vi "TCP client test.vi"() -> ()   [LabVIEW 2014]
panel:
  out "x-y":u32
  out "毫秒计时值":u32
  out "长度":i32
  out "服务器消息":string
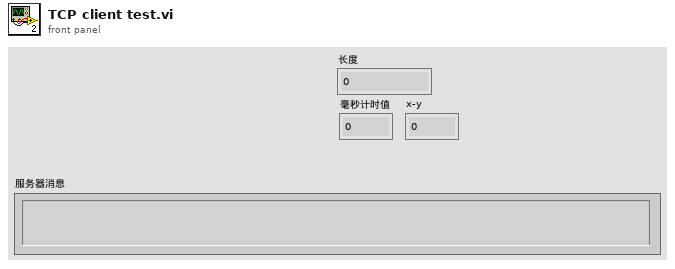
[diagram p1: front panel]
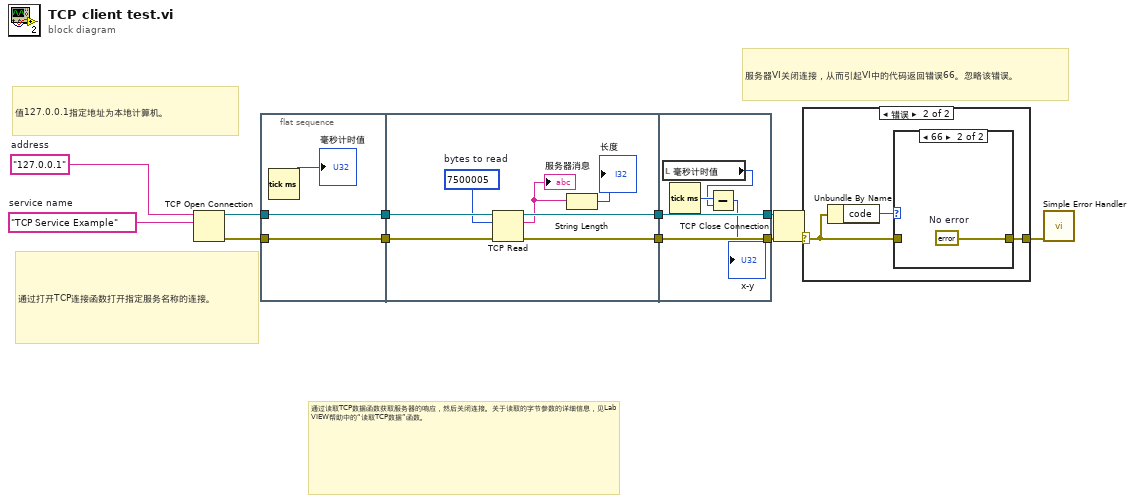
[diagram p0: block diagram]
diagram:
  w7 = "TCP Service Example"  # service name
  w8 = "127.0.0.1"  # address
  # "服务器VI关闭连接，从而引起VI中的代码返回错误66。忽略该错误。"
  # "值127.0.0.1指定地址为本地计算机。"
  # "通过打开TCP连接函数打开指定服务名称的连接。"
  # "通过读取TCP数据函数获取服务器的响应，然后关闭连接。关于读取的字节参数的详细信息，见LabVIEW帮助中的“读取TCP数据”函数。"
  n1 = TCP Open Connection(address=w8, remote port or service name=w7) -> (connection ID=w11:refnum<k5>, error out=w12:errorcluster)  [unwired: 3 in]
  n2 = flat-sequence {
    tunnel: w11 -> [w14]
    tunnel: w12 -> [w15]
    tunnel: [w15] -> w4
    tunnel: [w14] -> w3
    tunnel: w4 -> [w22]
    tunnel: w3 -> [w21]
    tunnel: [w20] -> w2
    tunnel: [w19] -> w1
    tunnel: [w26] -> w9
    tunnel: [w27] -> w10
    tunnel: w2 -> [w27]
    tunnel: w1 -> [w26]
    frame #0 {
      n3 = Tick Count (ms)() -> (millisecond timer value=→"毫秒计时值":u32)
    }
    frame #1 {
      w18 = 7500005  # bytes to read
      n4 = TCP Read(connection ID=w21, bytes to read=w18, error in (no error)=w22) -> (connection ID out=w20:refnum<k5>, data out=w17:string, error out=w19:errorcluster)  [unwired: 2 in]
      "服务器消息" <- w17
      n5 = String Length(string=w17) -> (length=→"长度":i32)
    }
    frame #2 {
      n6 = local read "毫秒计时值"() -> (w24:u32)
      n7 = Tick Count (ms)() -> (millisecond timer value=w25:u32)
      n8 = Subtract(x=w25, y=w24) -> (x-y=→"x-y":u32)
    }
  }
  n9 = TCP Close Connection(connection ID=w10, error in (no error)=w9) -> (error out=w6:errorcluster)  [unwired: 1 in, 1 out]
  n10 = case shown="错误" w6 {
    selector: w6 -> [w28 w30]
    tunnel: [w28 w29] -> w5
    frame No Error {
    }
    frame Error {
      n11 = Unbundle By Name(w30) -> ("code"=w31:i32)
      n12 = case shown="66" w31 {
        tunnel: w30 -> [w32 _]
        tunnel: [w32 w33] -> w29
        frame Default {
        }
        frame 66 {
          w33 = errorcluster {"status"=FALSE, "code"=0, "source"=""}  # No error
        }
      }
    }
  }
  n13 = call <vilib>:"Simple Error Handler.vi"("error in (no error)"=w5) -> ()  [unwired: 4 in, 5 out]
